vi "Configure Standard Waveform Advanced (Pulse).vi"(4 "Pulse Duty Cycle (10 Percent)":dbl=10.0, 5 "Pulse Width (100 us)":dbl=0.0001, 6 "Trail Edge (10 ns)":dbl=10.0, 7 "Lead Edge (10 ns)":dbl=10.0, 8 "error in (no error)":errorcluster, 9 "Pulse Variable To Held Const(0: Width)":i32(ring) items=["Width", "Duty Cycle"], 10 "Channel (1: 1)":i32(ring)=1 items=["1"=1, "2"=2], 11 "VISA resource name":refnum<visa-resource-name>) -> (0 "error out":errorcluster, 3 "VISA resource name out":refnum<visa-resource-name>)   [LabVIEW 2016, in "Agilent 3352X Series.lvlib"]
doc: "Provides Configurations for pulse waveform"
uses:
  Agilent 3352X Series.lvlib
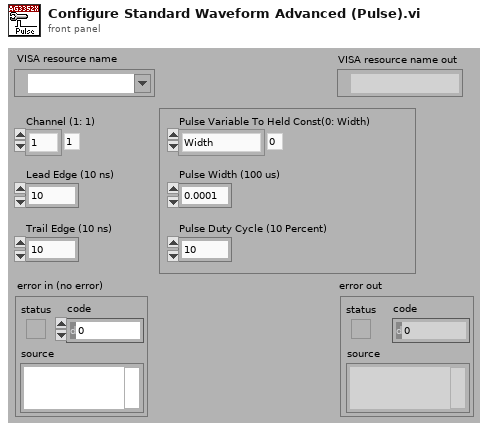
[diagram p1: front panel]
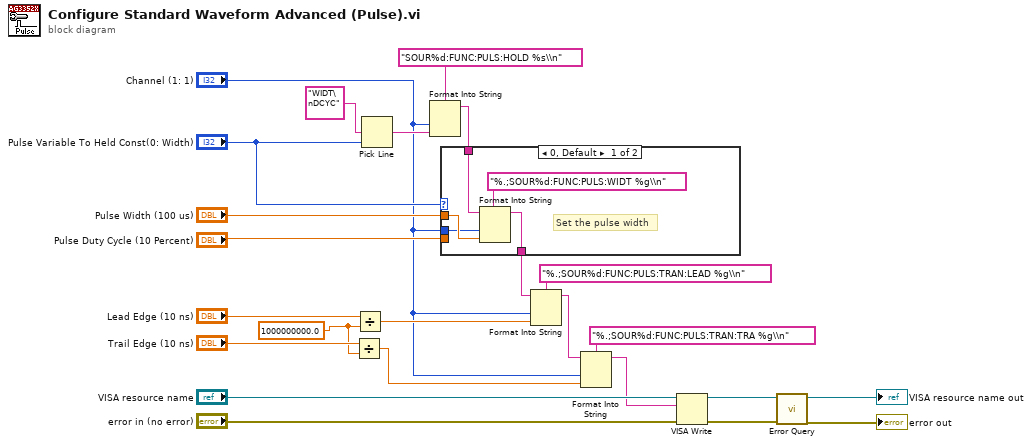
[diagram p0: block diagram]
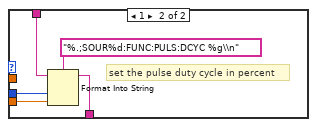
[diagram p2: hidden frame]
diagram:
  w8 = 1000000000.0 ("y")
  n1 = Divide(x="Trail Edge (10 ns)", y=w8) -> (x/y=w3:dbl)
  n2 = Divide(x="Lead Edge (10 ns)", y=w8) -> (x/y=w10:dbl)
  n3 = Pick Line(multi-line string="WIDT\nDCYC", line index="Pulse Variable To Held Const(0: Width)") -> (output string=w21:string)  [unwired: 1 out]
  n4 = Format Into String(format string="SOUR%d:FUNC:PULS:HOLD %s\\n", "Channel (1: 1)", w21) -> (resulting string=w6:string)  [unwired: 2 in, 1 out]
  n5 = case shown="0, Default" "Pulse Variable To Held Const(0: Width)" {
    tunnel: "Channel (1: 1)" -> [w25 w33]
    tunnel: "Pulse Duty Cycle (10 Percent)" -> [_ w32]
    tunnel: [w26 w31] -> w7
    tunnel: w6 -> [w28 w30]
    tunnel: "Pulse Width (100 us)" -> [w29 _]
    frame 0, Default {
      # "Set the pulse width"
      n6 = Format Into String(format string="%.;SOUR%d:FUNC:PULS:WIDT %g\\n", initial string=w28, w25, w29) -> (resulting string=w26:string)  [unwired: 1 in, 1 out]
    }
    frame 1 {
      # "set the pulse duty cycle in percent"
      n7 = Format Into String(format string="%.;SOUR%d:FUNC:PULS:DCYC %g\\n", initial string=w30, w33, w32) -> (resulting string=w31:string)  [unwired: 1 in, 1 out]
    }
  }
  n8 = Format Into String(format string="%.;SOUR%d:FUNC:PULS:TRAN:LEAD %g\\n", initial string=w7, "Channel (1: 1)", w10) -> (resulting string=w19:string)  [unwired: 1 in, 1 out]
  n9 = Format Into String(format string="%.;SOUR%d:FUNC:PULS:TRAN:TRA %g\\n", initial string=w19, "Channel (1: 1)", w3) -> (resulting string=w1:string)  [unwired: 1 in, 1 out]
  n10 = VISA Write(VISA resource name="VISA resource name", write buffer=w1, error in (no error)="error in (no error)") -> (VISA resource name out=w15:refnum<visa-resource-name>, error out=w14:errorcluster)  [unwired: 1 out]
  n11 = call "Error Query.vi"("error in (no error)"=w14, "VISA resource name"=w15) -> ("error out"=→"error out":errorcluster, "VISA resource name out"=→"VISA resource name out":refnum<visa-resource-name>)  [unwired: 8 out]
